vi "Check Hysteresis.vi"(9 "State In":T2, 10 "Threshold Settings":T1={"threshold"=0.0, "hysteresis"=0.0, "slope (rising)"=enum."rising"}, 11 "Analog Tach Signal":fxp<+/-,24,4>) -> (1 "State Out":T2, 2 "Event Occurred?":bool)   [LabVIEW 2014, in "Tachometer (SGL).lvlib"]
uses:
  Tachometer (SGL).lvlib
  Tach State.ctl
  Threshold Settings.ctl
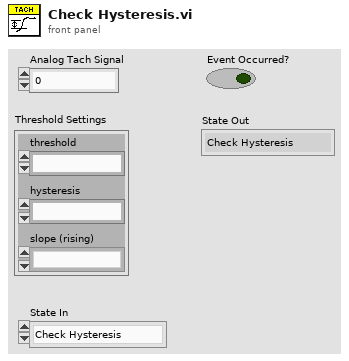
[diagram p1: front panel]
types:
  T1 = typedef "Tachometer (SGL).lvlib/Threshold Settings.ctl" = cluster{"threshold":fxp<+/-,24,4>, "hysteresis":fxp<+/-,24,4>, "slope (rising)":enum16{"falling", "rising"}}
  T2 = typedef "Tachometer (SGL).lvlib/Tach State.ctl" = enum16{"Check Hysteresis", "Check Threshold"}
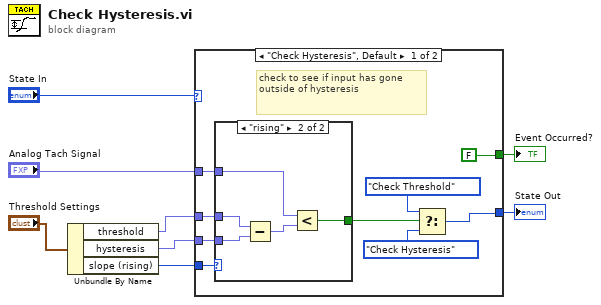
[diagram p0: block diagram]
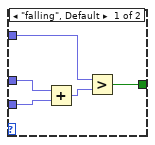
[diagram p2: hidden frame]
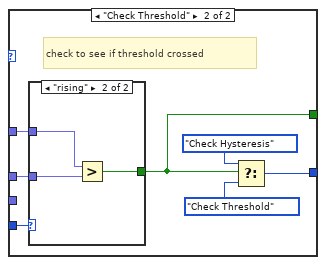
[diagram p3: hidden frame]
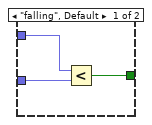
[diagram p4: hidden frame]
diagram:
  n1 = Unbundle By Name("Threshold Settings") -> ("threshold"=w3:fxp<+/-,24,4>, "hysteresis"=w2:fxp<+/-,24,4>, "slope (rising)"=w1:enum16{"falling", "rising"})
  n2 = case shown="\"Check Hysteresis\", Default" "State In" {
    tunnel: [w10 w29] -> w7
    tunnel: "Analog Tach Signal" -> [w16 w33]
    tunnel: w1 -> [w17 w34]
    tunnel: w3 -> [w15 w32]
    tunnel: w2 -> [w14 _]
    tunnel: [FALSE w28] -> w5
    frame "Check Hysteresis", Default {
      # "check to see if input has gone outside of hysteresis"
      n3 = case shown="\"rising\"" w17 {
        tunnel: w16 -> [w20 w24]
        tunnel: w15 -> [w22 w26]
        tunnel: w14 -> [w21 w27]
        tunnel: [w18 w23] -> w13
        frame "falling", Default {
          n4 = Add(x=w22, y=w21) -> (x+y=w19:fxp<+/-,25,5>)
          n5 = Greater?(x=w20, y=w19) -> (0:w18:bool)
        }
        frame "rising" {
          n6 = Subtract(x=w26, y=w27) -> (x-y=w25:fxp<+/-,25,5>)
          n7 = Less?(x=w24, y=w25) -> (x < y?=w23:bool)
        }
      }
      n8 = Select(t=Tach_State."Check Threshold" ("state"), s=w13, f=Tach_State."Check Hysteresis" ("state")) -> (s? t:f=w10:T2)
    }
    frame "Check Threshold" {
      # "check to see if threshold crossed"
      n9 = case shown="\"rising\"" w34 {
        tunnel: w33 -> [w37 w40]
        tunnel: w32 -> [w35 w38]
        tunnel: [w36 w39] -> w28
        frame "falling", Default {
          n10 = Less?(x=w37, y=w35) -> (x < y?=w36:bool)
        }
        frame "rising" {
          n11 = Greater?(x=w40, y=w38) -> (0:w39:bool)
        }
      }
      n12 = Select(t=Tach_State."Check Hysteresis" ("state"), s=w28, f=Tach_State."Check Threshold" ("state")) -> (s? t:f=w29:T2)
    }
  }
  "State Out" <- w7
  "Event Occurred?" <- w5
